vi "EditorPDF stateMachine.vi"(7 "state":T5(ring), 8 "error in (no error)":errorcluster, 10 "Parameter":T3={"Details"={"Title"="", "Subject"="", "Keywords"="", "Author"=""}, "Header/Footer"={"Header"="", "Footer"=""}, "Standard Page"={"Page Size"=10, "Portrait (T:Yes)"=TRUE}} {"Standard Page"."Page Size" items=["LETTER", "NOTE", "LEGAL", "TABLOID", "EXECUTIVE", "POSTCARD", "A0", "A1", "A2", "A3", "A4", "A5", "A6", "A7", "A8", "A9", "A10", "B0", "B1", "B2", "B3", "B4", "B5", "B6", "B7", "B8", "B9", "B10", "ARCH_E", "ARCH_D", "ARCH_C", "ARCH_B", "ARCH_A", "FLSA", "FLSE", "HALFLETTER", "_11X17", "ID_1", "ID_2", "ID_3", "LEDGER", "CROWN_QUARTO", "LARGE_CROWN_QUARTO", "DEMY_QUARTO", "ROYAL_QUARTO", "CROWN_OCTAVO", "LARGE_CROWN_OCTAVO", "DEMY_OCTAVO", "ROYAL_OCTAVO", "SMALL_PAPERBACK", "PENGUIN_SMALL_PAPERBACK", "PENGUIN_LARGE_PAPERBACK"]}, 11 "Refnum":T4) -> (0 "error out":errorcluster)   [LabVIEW 2018, in "CreatePDF.lvclass"]
uses:
  CreatePDF.lvclass
  <vilib>/Simplicity AI/SAI_PDF_API/Classes/Context/Controls/SAI_PDF_StdPageLayout.ctl
  <vilib>/Simplicity AI/SAI_PDF_API/Classes/Context/Controls/SAI_PDF_StdPageSize.ctl
  <vilib>/Simplicity AI/SAI_PDF_API/Classes/Context/Context.lvclass
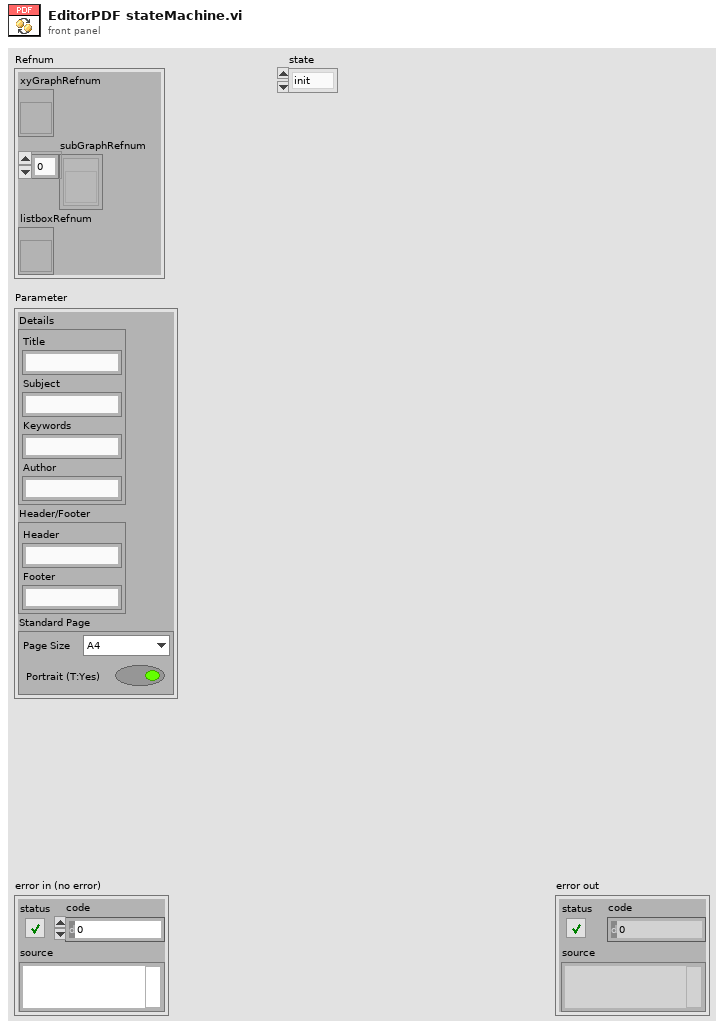
[diagram p1: front panel]
types:
  T1 = typedef "SAI_PDF_Toolkit.lvlib/Context.lvclass/SAI_PDF_StdPageLayout.ctl" = cluster{"Page Size":T2, "Portrait (T:Yes)":bool}
  T2 = typedef "SAI_PDF_Toolkit.lvlib/Context.lvclass/SAI_PDF_StdPageSize.ctl" = i32
  T3 = cluster{"Details":cluster{"Title":string, "Subject":string, "Keywords":string, "Author":string}, "Header/Footer":cluster{"Header":string, "Footer":string}, "Standard Page":T1}
  T4 = cluster{"xyGraphRefnum":refnum<vi>, "subGraphRefnum":refnum<vi>[], "listboxRefnum":refnum<vi>}
  T5 = enum16{"init", "setRefnum", "setParam", "create"}
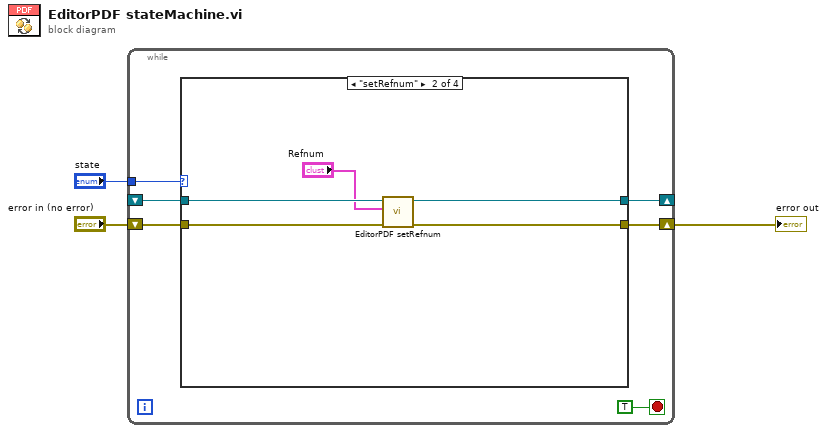
[diagram p0: block diagram]
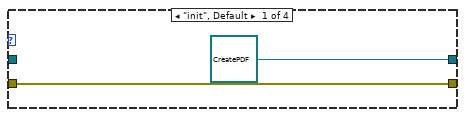
[diagram p2: hidden frame]
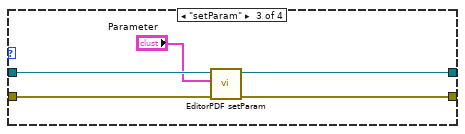
[diagram p3: hidden frame]
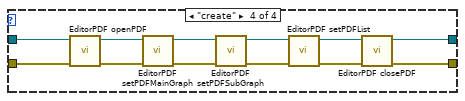
[diagram p4: hidden frame]
diagram:
  n1 = while {
    tunnel: "state" -> [w8]
    shift-right: [w7] -> _
    shift-left: _ -> [w6]
    shift-right: [w5] -> w2
    shift-left: "error in (no error)" -> [w4]
    stop <- TRUE stop-if-true
    n2 = case shown="\"setRefnum\"" w8 {
      tunnel: [refnum<class "CreatePDF.lvclass"> refnum ("CreatePDF.lvclass") w15 w19 w22] -> w7
      tunnel: w6 -> [_ w16 w21 w25]
      tunnel: [w10 w14 w18 w23] -> w5
      tunnel: w4 -> [w10 w13 w17 w24]
      frame "init", Default {
      }
      frame "setRefnum" {
        n3 = call "EditorPDF setRefnum.vi"("error in (no error)"=w13, "Refnum"="Refnum", "CreatePDF in"=w16) -> ("error out"=w14:errorcluster, "CreatePDF out"=w15:refnum<class "CreatePDF.lvclass">)  [unwired: 7 in]
      }
      frame "setParam" {
        n4 = call "EditorPDF setParam.vi"("error in (no error)"=w17, "Parameter"="Parameter", "CreatePDF in"=w21) -> ("error out"=w18:errorcluster, "CreatePDF out"=w19:refnum<class "CreatePDF.lvclass">)  [unwired: 7 in]
      }
      frame "create" {
        n5 = call "EditorPDF openPDF.vi"("error in (no error)"=w24, "CreatePDF in"=w25) -> ("error out"=w33:errorcluster, "CreatePDF out"=w26:refnum<class "CreatePDF.lvclass">)  [unwired: 8 in]
        n6 = call "EditorPDF setPDFMainGraph.vi"("error in (no error)"=w33, "CreatePDF in"=w26) -> ("error out"=w32:errorcluster, "CreatePDF out"=w27:refnum<class "CreatePDF.lvclass">)  [unwired: 8 in]
        n7 = call "EditorPDF setPDFSubGraph.vi"("error in (no error)"=w32, "CreatePDF in"=w27) -> ("error out"=w31:errorcluster, "CreatePDF out"=w28:refnum<class "CreatePDF.lvclass">)  [unwired: 8 in]
        n8 = call "EditorPDF setPDFList.vi"("error in (no error)"=w31, "CreatePDF in"=w28) -> ("error out"=w30:errorcluster, "CreatePDF out"=w29:refnum<class "CreatePDF.lvclass">)  [unwired: 8 in]
        n9 = call "EditorPDF closePDF.vi"("error in (no error)"=w30, "CreatePDF in"=w29) -> ("error out"=w23:errorcluster, "CreatePDF out"=w22:refnum<class "CreatePDF.lvclass">)  [unwired: 8 in]
      }
    }
  }
  "error out" <- w2
